vi "Device ID.vi"(4 "Date (YYYYMMDD)":string, 5 "Sample (SAXXXX)":string) -> (1 "Device ID":string)   [LabVIEW 2019, in "Control Experiment.lvclass"]
uses:
  Control Experiment.lvclass
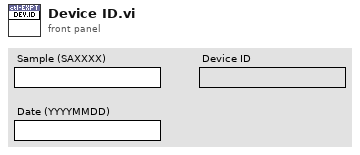
[diagram p1: front panel]
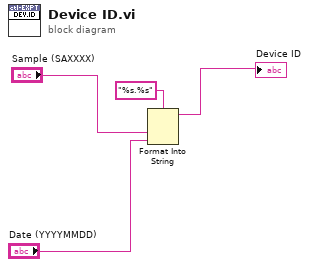
[diagram p0: block diagram]
diagram:
  n1 = Format Into String(format string="%s.%s", "Sample (SAXXXX)", "Date (YYYYMMDD)") -> (resulting string=→"Device ID":string)  [unwired: 2 in, 1 out]
